vi "GlobalGetMesaurementStatus.vi"() -> ()   [LabVIEW 2013]
panel:
  out "FifoMesaurementTerminatior":bool
  out "MeasurementAktiv":bool
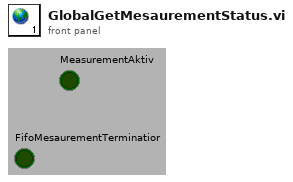
[diagram p1: front panel]
diagram:
